vi "HandleObservationSync.vi"(8 "error in (no error)":errorcluster, 11 "S4GUI in":refnum<class "S4GUI.lvclass">) -> (0 "error out":errorcluster, 3 "S4GUI out":refnum<class "S4GUI.lvclass">)   [LabVIEW 2018, in "S4GUI.lvclass"] (continued)
          # "Espera terminar o envio de WAIT EXPOSE COMMAND para todos os ACS."
          n1279 = call-dynamic "VerifyAcqIdle.vi"("error in (no error)"=w3504, "S4GUI in"=w3503) -> ("error out"=w3509:errorcluster, "idle"=w3508:bool, "S4GUI out"=w3510:refnum<class "S4GUI.lvclass">)  [unwired: 6 in, 1 out]
          n1280 = disable-structure shown="Enabled" {
            disable-tunnel: w3506 -> [w3513 _]
            disable-tunnel: [w3512 u32 325] -> w3505
            frame Disabled {
              n1281 = Increment(x=w3513) -> (x+1=w3512:u32)
            }
            frame Enabled {
            }
          }
          n1282 = Select(t=w3505, s=w3508, f=w3506) -> (s? t:f=w3507:u32)
          n1283 = Bundle By Name(cluster=w3510, "Obs_state"=w3507) -> (w3511:refnum<class "S4GUI.lvclass">)
        }
        frame 323 {
          n1284 = call-dynamic "Read AcquisitionA.vi"("error in (no error)"=w3577, "S4ACS_GUI in"=w3578) -> ("error out"=w3532:errorcluster, "Acquisition.lvclass"=w3533:refnum<class "Acquisition.lvclass">, "S4ACS_GUI out"=w3580:refnum<class "S4GUI.lvclass">)  [unwired: 7 in]
          n1285 = call-dynamic "Read enabled.vi"("error in (no error)"=w3532, "Server in"=w3533) -> ("error out"=w3531:errorcluster, "enabled"=w3518:bool, "Server out"=w3534:refnum<class "Acquisition.lvclass">)  [unwired: 7 in]
          n1286 = call "Read connection.vi"("error in (no error)"=w3531, "Server in"=w3534) -> ("error out"=w3557:errorcluster, "connection"=w3541:bool, "Server out"=w3558:refnum<class "Acquisition.lvclass">)  [unwired: 7 in]
          n1287 = And(x=w3541, y=w3518) -> (x .and. y?=w3542:bool)
          n1288 = case shown="True" w3542 {
            tunnel: w3558 -> [w3687 w3703]
            tunnel: w3557 -> [w3686 w3702]
            tunnel: [w3687 w3700] -> w3581
            tunnel: [w3686 w3699] -> w3579
            tunnel: [w3683 u32 0 ("New_State")] -> w3547
            tunnel: w3518 -> [w3682 _]
            frame False {
              n1289 = Select(t=u32 1, s=w3682, f=u32 0) -> (s? t:f=w3683:u32)
            }
            frame True {
              n1290 = call-dynamic "Read Channel.vi"("error in (no error)"=w3702, "Acquisition in"=w3703) -> ("error out"=w3695:errorcluster, "Channel.lvclass"=w3694:refnum<class "Channel.lvclass">, "Acquisition out"=w3701:refnum<class "Acquisition.lvclass">)  [unwired: 7 in]
              n1291 = call-dynamic "Read State Machine.vi"("error in (no error)"=w3695, "Device in"=w3694) -> ("error out"=w3696:errorcluster, "State Machine.lvclass"=w3698:refnum<class "State Machine.lvclass">, "Device out"=w3692:refnum<class "Channel.lvclass">)  [unwired: 7 in]
              n1292 = call "Next State.vi"("error in (no error)"=w3696, "New_State"=50, "State Machine in"=w3698) -> ("error out"=w3689:errorcluster, "State Machine out"=w3690:refnum<class "State Machine.lvclass">)  [unwired: 7 in]
              n1293 = call-dynamic "Write State Machine.vi"("error in (no error)"=w3689, "State Machine.lvclass"=w3690, "Device in"=w3692) -> ("error out"=w3691:errorcluster, "Device out"=w3693:refnum<class "Channel.lvclass">)  [unwired: 7 in]
              n1294 = call-dynamic "Write Channel.vi"("error in (no error)"=w3691, "Channel.lvclass"=w3693, "Acquisition in"=w3701) -> ("error out"=w3699:errorcluster, "Acquisition out"=w3700:refnum<class "Acquisition.lvclass">)  [unwired: 7 in]
            }
          }
          n1295 = call-dynamic "Write AcquisitionA.vi"("error in (no error)"=w3579, "Acquisition.lvclass"=w3581, "S4ACS_GUI in"=w3580) -> ("error out"=w3574:errorcluster, "S4ACS_GUI out"=w3575:refnum<class "S4GUI.lvclass">)  [unwired: 7 in]
          n1296 = call "Read AcquisitionB.vi"("error in (no error)"=w3574, "S4ACS_GUI in"=w3575) -> ("error out"=w3528:errorcluster, "Acquisition.lvclass"=w3530:refnum<class "Acquisition.lvclass">, "S4ACS_GUI out"=w3572:refnum<class "S4GUI.lvclass">)  [unwired: 7 in]
          n1297 = call-dynamic "Read enabled.vi"("error in (no error)"=w3528, "Server in"=w3530) -> ("error out"=w3527:errorcluster, "enabled"=w3517:bool, "Server out"=w3529:refnum<class "Acquisition.lvclass">)  [unwired: 7 in]
          n1298 = call "Read connection.vi"("error in (no error)"=w3527, "Server in"=w3529) -> ("error out"=w3555:errorcluster, "connection"=w3539:bool, "Server out"=w3556:refnum<class "Acquisition.lvclass">)  [unwired: 7 in]
          n1299 = And(x=w3539, y=w3517) -> (x .and. y?=w3540:bool)
          n1300 = case shown="True" w3540 {
            tunnel: w3556 -> [w3665 w3681]
            tunnel: w3555 -> [w3664 w3680]
            tunnel: [w3665 w3678] -> w3573
            tunnel: [w3664 w3677] -> w3571
            tunnel: [w3661 u32 0 ("New_State")] -> w3546
            tunnel: w3517 -> [w3660 _]
            frame False {
              n1301 = Select(t=u32 2, s=w3660, f=u32 0) -> (s? t:f=w3661:u32)
            }
            frame True {
              n1302 = call-dynamic "Read Channel.vi"("error in (no error)"=w3680, "Acquisition in"=w3681) -> ("error out"=w3673:errorcluster, "Channel.lvclass"=w3672:refnum<class "Channel.lvclass">, "Acquisition out"=w3679:refnum<class "Acquisition.lvclass">)  [unwired: 7 in]
              n1303 = call-dynamic "Read State Machine.vi"("error in (no error)"=w3673, "Device in"=w3672) -> ("error out"=w3674:errorcluster, "State Machine.lvclass"=w3676:refnum<class "State Machine.lvclass">, "Device out"=w3670:refnum<class "Channel.lvclass">)  [unwired: 7 in]
              n1304 = call "Next State.vi"("error in (no error)"=w3674, "New_State"=50, "State Machine in"=w3676) -> ("error out"=w3667:errorcluster, "State Machine out"=w3668:refnum<class "State Machine.lvclass">)  [unwired: 7 in]
              n1305 = call-dynamic "Write State Machine.vi"("error in (no error)"=w3667, "State Machine.lvclass"=w3668, "Device in"=w3670) -> ("error out"=w3669:errorcluster, "Device out"=w3671:refnum<class "Channel.lvclass">)  [unwired: 7 in]
              n1306 = call-dynamic "Write Channel.vi"("error in (no error)"=w3669, "Channel.lvclass"=w3671, "Acquisition in"=w3679) -> ("error out"=w3677:errorcluster, "Acquisition out"=w3678:refnum<class "Acquisition.lvclass">)  [unwired: 7 in]
            }
          }
          n1307 = call "Write AcquisitionB.vi"("error in (no error)"=w3571, "Acquisition.lvclass"=w3573, "S4ACS_GUI in"=w3572) -> ("error out"=w3567:errorcluster, "S4ACS_GUI out"=w3566:refnum<class "S4GUI.lvclass">)  [unwired: 7 in]
          n1308 = call-dynamic "Read AcquisitionC.vi"("error in (no error)"=w3567, "S4ACS_GUI in"=w3566) -> ("error out"=w3524:errorcluster, "Acquisition.lvclass"=w3526:refnum<class "Acquisition.lvclass">, "S4ACS_GUI out"=w3569:refnum<class "S4GUI.lvclass">)  [unwired: 7 in]
          n1309 = call-dynamic "Read enabled.vi"("error in (no error)"=w3524, "Server in"=w3526) -> ("error out"=w3523:errorcluster, "enabled"=w3516:bool, "Server out"=w3525:refnum<class "Acquisition.lvclass">)  [unwired: 7 in]
          n1310 = call "Read connection.vi"("error in (no error)"=w3523, "Server in"=w3525) -> ("error out"=w3553:errorcluster, "connection"=w3536:bool, "Server out"=w3554:refnum<class "Acquisition.lvclass">)  [unwired: 7 in]
          n1311 = And(x=w3536, y=w3516) -> (x .and. y?=w3538:bool)
          n1312 = case shown="True" w3538 {
            tunnel: [w3642 w3651] -> w3570
            tunnel: [w3643 w3650] -> w3568
            tunnel: w3554 -> [w3643 w3648]
            tunnel: w3553 -> [w3642 w3647]
            tunnel: [w3639 u32 0 ("New_State")] -> w3545
            tunnel: w3516 -> [w3638 _]
            frame False {
              n1313 = Select(t=u32 4, s=w3638, f=u32 0) -> (s? t:f=w3639:u32)
            }
            frame True {
              n1314 = call-dynamic "Read Channel.vi"("error in (no error)"=w3647, "Acquisition in"=w3648) -> ("error out"=w3655:errorcluster, "Channel.lvclass"=w3656:refnum<class "Channel.lvclass">, "Acquisition out"=w3649:refnum<class "Acquisition.lvclass">)  [unwired: 7 in]
              n1315 = call-dynamic "Read State Machine.vi"("error in (no error)"=w3655, "Device in"=w3656) -> ("error out"=w3654:errorcluster, "State Machine.lvclass"=w3652:refnum<class "State Machine.lvclass">, "Device out"=w3658:refnum<class "Channel.lvclass">)  [unwired: 7 in]
              n1316 = call "Next State.vi"("error in (no error)"=w3654, "New_State"=50, "State Machine in"=w3652) -> ("error out"=w3646:errorcluster, "State Machine out"=w3645:refnum<class "State Machine.lvclass">)  [unwired: 7 in]
              n1317 = call-dynamic "Write State Machine.vi"("error in (no error)"=w3646, "State Machine.lvclass"=w3645, "Device in"=w3658) -> ("error out"=w3659:errorcluster, "Device out"=w3657:refnum<class "Channel.lvclass">)  [unwired: 7 in]
              n1318 = call-dynamic "Write Channel.vi"("error in (no error)"=w3659, "Channel.lvclass"=w3657, "Acquisition in"=w3649) -> ("error out"=w3651:errorcluster, "Acquisition out"=w3650:refnum<class "Acquisition.lvclass">)  [unwired: 7 in]
            }
          }
          n1319 = call-dynamic "Write AcquisitionC.vi"("error in (no error)"=w3570, "Acquisition.lvclass"=w3568, "S4ACS_GUI in"=w3569) -> ("error out"=w3564:errorcluster, "S4ACS_GUI out"=w3563:refnum<class "S4GUI.lvclass">)  [unwired: 7 in]
          n1320 = call-dynamic "Read AcquisitionD.vi"("error in (no error)"=w3564, "S4ACS_GUI in"=w3563) -> ("error out"=w3520:errorcluster, "Acquisition.lvclass"=w3522:refnum<class "Acquisition.lvclass">, "S4ACS_GUI out"=w3562:refnum<class "S4GUI.lvclass">)  [unwired: 7 in]
          n1321 = call-dynamic "Read enabled.vi"("error in (no error)"=w3520, "Server in"=w3522) -> ("error out"=w3519:errorcluster, "enabled"=w3515:bool, "Server out"=w3521:refnum<class "Acquisition.lvclass">)  [unwired: 7 in]
          n1322 = call "Read connection.vi"("error in (no error)"=w3519, "Server in"=w3521) -> ("error out"=w3551:errorcluster, "connection"=w3535:bool, "Server out"=w3552:refnum<class "Acquisition.lvclass">)  [unwired: 7 in]
          n1323 = And(x=w3535, y=w3515) -> (x .and. y?=w3537:bool)
          n1324 = case shown="True" w3537 {
            tunnel: w3551 -> [w3620 w3637]
            tunnel: [w3620 w3636] -> w3565
            tunnel: w3552 -> [w3621 w3627]
            tunnel: [w3621 w3625] -> w3561
            tunnel: [w3617 u32 0 ("New_State")] -> w3544
            tunnel: w3515 -> [w3616 _]
            frame False {
              n1325 = Select(t=u32 8, s=w3616, f=u32 0) -> (s? t:f=w3617:u32)
            }
            frame True {
              n1326 = call-dynamic "Read Channel.vi"("error in (no error)"=w3637, "Acquisition in"=w3627) -> ("error out"=w3632:errorcluster, "Channel.lvclass"=w3631:refnum<class "Channel.lvclass">, "Acquisition out"=w3626:refnum<class "Acquisition.lvclass">)  [unwired: 7 in]
              n1327 = call-dynamic "Read State Machine.vi"("error in (no error)"=w3632, "Device in"=w3631) -> ("error out"=w3633:errorcluster, "State Machine.lvclass"=w3635:refnum<class "State Machine.lvclass">, "Device out"=w3629:refnum<class "Channel.lvclass">)  [unwired: 7 in]
              n1328 = call "Next State.vi"("error in (no error)"=w3633, "New_State"=50, "State Machine in"=w3635) -> ("error out"=w3623:errorcluster, "State Machine out"=w3624:refnum<class "State Machine.lvclass">)  [unwired: 7 in]
              n1329 = call-dynamic "Write State Machine.vi"("error in (no error)"=w3623, "State Machine.lvclass"=w3624, "Device in"=w3629) -> ("error out"=w3628:errorcluster, "Device out"=w3630:refnum<class "Channel.lvclass">)  [unwired: 7 in]
              n1330 = call-dynamic "Write Channel.vi"("error in (no error)"=w3628, "Channel.lvclass"=w3630, "Acquisition in"=w3626) -> ("error out"=w3636:errorcluster, "Acquisition out"=w3625:refnum<class "Acquisition.lvclass">)  [unwired: 7 in]
            }
          }
          n1331 = call-dynamic "Write AcquisitionD.vi"("error in (no error)"=w3565, "Acquisition.lvclass"=w3561, "S4ACS_GUI in"=w3562) -> ("error out"=w3560:errorcluster, "S4ACS_GUI out"=w3559:refnum<class "S4GUI.lvclass">)  [unwired: 7 in]
          n1332 = Compound Arithmetic op=ADD(w3547, w3546, w3545, w3544) -> (w3548:u32)
          n1333 = case shown="0, Default" w3548 {
            tunnel: w3543 -> [w3585 _ _ _ _ _ _ _ _ _ _ _ _ _ _ _]
            tunnel: [w3584 u32 1 ("Obs_state") u32 1 ("Obs_state") u32 1 ("Obs_state") u32 1 ("Obs_state") u32 1 ("Obs_state") u32 1 ("Obs_state") u32 1 ("Obs_state") u32 1 ("Obs_state") u32 1 ("Obs_state") u32 1 ("Obs_state") u32 1 ("Obs_state") u32 1 ("Obs_state") u32 1 ("Obs_state") u32 1 ("Obs_state") u32 1 ("Obs_state")] -> w3549
            tunnel: ["" ("Error Msg") "ERROR: Lost channel 1 connection... - HandleObservationSync.vi state 323" ("Error Msg") "ERROR: Lost channel 2 connection...- HandleObservationSync.vi state 323" ("Error Msg") "ERROR: Lost channels 1 and 2 connection...- HandleObservationSync.vi state 323" ("Error Msg") "ERROR: Lost channel 3 connection...- HandleObservationSync.vi state 323" ("Error Msg") "ERROR: Lost channels 1 and  3 connection...- HandleObservationSync.vi state 323" ("Error Msg") "ERROR:  Lost channels 2 and  3 connection...- HandleObservationSync.vi state 323" ("Error Msg") "ERROR:  Lost channels 1, 2 and  3 connection...- HandleObservationSync.vi state 323" ("Error Msg") "ERROR: Lost channel 4 connection...- HandleObservationSync.vi state 323" ("Error Msg") "ERROR:  Lost channels 1 and 4 connection...- HandleObservationSync.vi state 323" ("Error Msg") "ERROR:  Lost channels 2 and 4 connection...- HandleObservationSync.vi state 323" ("Error Msg") "ERROR: Lost channels 1, 2 and 4 connection...- HandleObservationSync.vi state 323" ("Error Msg") "ERROR: Lost channels 3 and 4 connection...- HandleObservationSync.vi state 323" ("Error Msg") "ERROR: Lost channels 1, 3 and 4 connection...- HandleObservationSync.vi state 323" ("Error Msg") "ERROR: Lost channels 2, 3 and 4 connection...- HandleObservationSync.vi state 323" ("Error Msg") "ERROR: Lost channels 1, 2, 3 and 4 connection...- HandleObservationSync.vi state 323" ("Error Msg")] -> w3550
            frame 0, Default {
              n1334 = Increment(x=w3585) -> (x+1=w3584:u32)
              n1335 = Tick Count (ms)() -> (millisecond timer value=w3582:u32)
              n1336 = local write "time1"(w3582) -> ()
            }
            frame 1 {
            }
            frame 2 {
            }
            frame 3 {
            }
            frame 4 {
            }
            frame 5 {
            }
            frame 6 {
            }
            frame 7 {
            }
            frame 8 {
            }
            frame 9 {
            }
            frame 10 {
            }
            frame 11 {
            }
            frame 12 {
            }
            frame 13 {
            }
            frame 14 {
            }
            frame 15 {
            }
          }
          n1337 = Bundle By Name(cluster=w3559, "Obs_state"=w3549, "Error Msg"=w3550) -> (w3576:refnum<class "S4GUI.lvclass">)
        }
        frame 324 {
          # "Espera terminar a execução do comando atual \nantes de ir ao proximo passo da Observação."
          n1338 = call-dynamic "Read AcquisitionA.vi"("error in (no error)"=w3757, "S4ACS_GUI in"=w3758) -> ("error out"=w3739:errorcluster, "Acquisition.lvclass"=w3740:refnum<class "Acquisition.lvclass">, "S4ACS_GUI out"=w3760:refnum<class "S4GUI.lvclass">)  [unwired: 7 in]
          n1339 = call "Read connection.vi"("error in (no error)"=w3739, "Server in"=w3740) -> ("error out"=w3738:errorcluster, "connection"=w3737:bool, "Server out"=w3736:refnum<class "Acquisition.lvclass">)  [unwired: 7 in]
          n1340 = case shown="True" w3737 {
            tunnel: w3738 -> [w3869 w3890]
            tunnel: [w3870 w3888] -> w3761
            tunnel: [w3869 w3887] -> w3759
            tunnel: [TRUE w3876] -> w3718
            tunnel: w3736 -> [w3870 w3879]
            tunnel: [FALSE w3871] -> w3716
            frame False {
            }
            frame True {
              n1341 = call-dynamic "Read Channel.vi"("error in (no error)"=w3890, "Acquisition in"=w3879) -> ("error out"=w3873:errorcluster, "Channel.lvclass"=w3875:refnum<class "Channel.lvclass">, "Acquisition out"=w3889:refnum<class "Acquisition.lvclass">)  [unwired: 7 in]
              n1342 = call-dynamic "Read wait_expose.vi"("error in (no error)"=w3873, "Channel in"=w3875) -> ("error out"=w3872:errorcluster, "wait_expose"=w3871:bool, "Channel out"=w3874:refnum<class "Channel.lvclass">)  [unwired: 7 in]
              n1343 = call-dynamic "Read State Machine.vi"("error in (no error)"=w3872, "Device in"=w3874) -> ("error out"=w3881:errorcluster, "State Machine.lvclass"=w3883:refnum<class "State Machine.lvclass">, "Device out"=w3885:refnum<class "Channel.lvclass">)  [unwired: 7 in]
              n1344 = call-dynamic "Read State.vi"("error in (no error)"=w3881, "State Machine in"=w3883) -> ("error out"=w3880:errorcluster, "State"=w3877:i32, "State Machine out"=w3882:refnum<class "State Machine.lvclass">)  [unwired: 7 in]
              n1345 = Greater?(x=w3877, y=53 ("x")) -> (0:w3876:bool)
              n1346 = call-dynamic "Write State Machine.vi"("error in (no error)"=w3880, "State Machine.lvclass"=w3882, "Device in"=w3885) -> ("error out"=w3884:errorcluster, "Device out"=w3886:refnum<class "Channel.lvclass">)  [unwired: 7 in]
              n1347 = call-dynamic "Write Channel.vi"("error in (no error)"=w3884, "Channel.lvclass"=w3886, "Acquisition in"=w3889) -> ("error out"=w3887:errorcluster, "Acquisition out"=w3888:refnum<class "Acquisition.lvclass">)  [unwired: 7 in]
            }
          }
          n1348 = call-dynamic "Write AcquisitionA.vi"("error in (no error)"=w3759, "Acquisition.lvclass"=w3761, "S4ACS_GUI in"=w3760) -> ("error out"=w3754:errorcluster, "S4ACS_GUI out"=w3753:refnum<class "S4GUI.lvclass">)  [unwired: 7 in]
          n1349 = call "Read AcquisitionB.vi"("error in (no error)"=w3754, "S4ACS_GUI in"=w3753) -> ("error out"=w3731:errorcluster, "Acquisition.lvclass"=w3735:refnum<class "Acquisition.lvclass">, "S4ACS_GUI out"=w3755:refnum<class "S4GUI.lvclass">)  [unwired: 7 in]
          n1350 = call "Read connection.vi"("error in (no error)"=w3731, "Server in"=w3735) -> ("error out"=w3732:errorcluster, "connection"=w3733:bool, "Server out"=w3734:refnum<class "Acquisition.lvclass">)  [unwired: 7 in]
          n1351 = case shown="True" w3733 {
            tunnel: w3732 -> [w3845 w3858]
            tunnel: w3734 -> [w3846 w3857]
            tunnel: [TRUE w3852] -> w3720
            tunnel: [w3845 w3856] -> w3752
            tunnel: [w3846 w3855] -> w3751
            tunnel: [FALSE w3847] -> w3715
            frame False {
            }
            frame True {
              n1352 = call-dynamic "Read Channel.vi"("error in (no error)"=w3858, "Acquisition in"=w3857) -> ("error out"=w3849:errorcluster, "Channel.lvclass"=w3851:refnum<class "Channel.lvclass">, "Acquisition out"=w3859:refnum<class "Acquisition.lvclass">)  [unwired: 7 in]
              n1353 = call-dynamic "Read wait_expose.vi"("error in (no error)"=w3849, "Channel in"=w3851) -> ("error out"=w3848:errorcluster, "wait_expose"=w3847:bool, "Channel out"=w3850:refnum<class "Channel.lvclass">)  [unwired: 7 in]
              n1354 = call-dynamic "Read State Machine.vi"("error in (no error)"=w3848, "Device in"=w3850) -> ("error out"=w3865:errorcluster, "State Machine.lvclass"=w3863:refnum<class "State Machine.lvclass">, "Device out"=w3861:refnum<class "Channel.lvclass">)  [unwired: 7 in]
              n1355 = call-dynamic "Read State.vi"("error in (no error)"=w3865, "State Machine in"=w3863) -> ("error out"=w3866:errorcluster, "State"=w3854:i32, "State Machine out"=w3864:refnum<class "State Machine.lvclass">)  [unwired: 7 in]
              n1356 = Greater?(x=w3854, y=53 ("x")) -> (0:w3852:bool)
              n1357 = call-dynamic "Write State Machine.vi"("error in (no error)"=w3866, "State Machine.lvclass"=w3864, "Device in"=w3861) -> ("error out"=w3862:errorcluster, "Device out"=w3860:refnum<class "Channel.lvclass">)  [unwired: 7 in]
              n1358 = call-dynamic "Write Channel.vi"("error in (no error)"=w3862, "Channel.lvclass"=w3860, "Acquisition in"=w3859) -> ("error out"=w3856:errorcluster, "Acquisition out"=w3855:refnum<class "Acquisition.lvclass">)  [unwired: 7 in]
            }
          }
          n1359 = call "Write AcquisitionB.vi"("error in (no error)"=w3752, "Acquisition.lvclass"=w3751, "S4ACS_GUI in"=w3755) -> ("error out"=w3744:errorcluster, "S4ACS_GUI out"=w3743:refnum<class "S4GUI.lvclass">)  [unwired: 7 in]
          n1360 = call-dynamic "Read AcquisitionC.vi"("error in (no error)"=w3744, "S4ACS_GUI in"=w3743) -> ("error out"=w3727:errorcluster, "Acquisition.lvclass"=w3730:refnum<class "Acquisition.lvclass">, "S4ACS_GUI out"=w3746:refnum<class "S4GUI.lvclass">)  [unwired: 7 in]
          n1361 = call "Read connection.vi"("error in (no error)"=w3727, "Server in"=w3730) -> ("error out"=w3726:errorcluster, "connection"=w3728:bool, "Server out"=w3729:refnum<class "Acquisition.lvclass">)  [unwired: 7 in]
          n1362 = case shown="True" w3728 {
            tunnel: [w3821 w3835] -> w3747
            tunnel: [w3822 w3834] -> w3745
            tunnel: w3726 -> [w3821 w3831]
            tunnel: w3729 -> [w3822 w3832]
            tunnel: [TRUE w3828] -> w3719
            tunnel: [FALSE w3823] -> w3714
            frame False {
            }
            frame True {
              n1363 = call-dynamic "Read Channel.vi"("error in (no error)"=w3831, "Acquisition in"=w3832) -> ("error out"=w3825:errorcluster, "Channel.lvclass"=w3827:refnum<class "Channel.lvclass">, "Acquisition out"=w3833:refnum<class "Acquisition.lvclass">)  [unwired: 7 in]
              n1364 = call-dynamic "Read wait_expose.vi"("error in (no error)"=w3825, "Channel in"=w3827) -> ("error out"=w3824:errorcluster, "wait_expose"=w3823:bool, "Channel out"=w3826:refnum<class "Channel.lvclass">)  [unwired: 7 in]
              n1365 = call-dynamic "Read State Machine.vi"("error in (no error)"=w3824, "Device in"=w3826) -> ("error out"=w3841:errorcluster, "State Machine.lvclass"=w3839:refnum<class "State Machine.lvclass">, "Device out"=w3837:refnum<class "Channel.lvclass">)  [unwired: 7 in]
              n1366 = call-dynamic "Read State.vi"("error in (no error)"=w3841, "State Machine in"=w3839) -> ("error out"=w3842:errorcluster, "State"=w3829:i32, "State Machine out"=w3840:refnum<class "State Machine.lvclass">)  [unwired: 7 in]
              n1367 = Greater?(x=w3829, y=53 ("x")) -> (0:w3828:bool)
              n1368 = call-dynamic "Write State Machine.vi"("error in (no error)"=w3842, "State Machine.lvclass"=w3840, "Device in"=w3837) -> ("error out"=w3838:errorcluster, "Device out"=w3836:refnum<class "Channel.lvclass">)  [unwired: 7 in]
              n1369 = call-dynamic "Write Channel.vi"("error in (no error)"=w3838, "Channel.lvclass"=w3836, "Acquisition in"=w3833) -> ("error out"=w3835:errorcluster, "Acquisition out"=w3834:refnum<class "Acquisition.lvclass">)  [unwired: 7 in]
            }
          }
          n1370 = call-dynamic "Write AcquisitionC.vi"("error in (no error)"=w3747, "Acquisition.lvclass"=w3745, "S4ACS_GUI in"=w3746) -> ("error out"=w3741:errorcluster, "S4ACS_GUI out"=w3742:refnum<class "S4GUI.lvclass">)  [unwired: 7 in]
          n1371 = call-dynamic "Read AcquisitionD.vi"("error in (no error)"=w3741, "S4ACS_GUI in"=w3742) -> ("error out"=w3722:errorcluster, "Acquisition.lvclass"=w3725:refnum<class "Acquisition.lvclass">, "S4ACS_GUI out"=w3748:refnum<class "S4GUI.lvclass">)  [unwired: 7 in]
          n1372 = call "Read connection.vi"("error in (no error)"=w3722, "Server in"=w3725) -> ("error out"=w3721:errorcluster, "connection"=w3723:bool, "Server out"=w3724:refnum<class "Acquisition.lvclass">)  [unwired: 7 in]
          n1373 = case shown="True" w3723 {
            tunnel: [w3798 w3818] -> w3750
            tunnel: [w3797 w3817] -> w3749
            tunnel: w3724 -> [w3798 w3816]
            tunnel: w3721 -> [w3797 w3815]
            tunnel: [TRUE w3804] -> w3717
            tunnel: [FALSE w3799] -> w3713
            frame False {
            }
            frame True {
              n1374 = call-dynamic "Read Channel.vi"("error in (no error)"=w3815, "Acquisition in"=w3816) -> ("error out"=w3801:errorcluster, "Channel.lvclass"=w3803:refnum<class "Channel.lvclass">, "Acquisition out"=w3814:refnum<class "Acquisition.lvclass">)  [unwired: 7 in]
              n1375 = call-dynamic "Read wait_expose.vi"("error in (no error)"=w3801, "Channel in"=w3803) -> ("error out"=w3800:errorcluster, "wait_expose"=w3799:bool, "Channel out"=w3802:refnum<class "Channel.lvclass">)  [unwired: 7 in]
              n1376 = call-dynamic "Read State Machine.vi"("error in (no error)"=w3800, "Device in"=w3802) -> ("error out"=w3808:errorcluster, "State Machine.lvclass"=w3810:refnum<class "State Machine.lvclass">, "Device out"=w3812:refnum<class "Channel.lvclass">)  [unwired: 7 in]
              n1377 = call-dynamic "Read State.vi"("error in (no error)"=w3808, "State Machine in"=w3810) -> ("error out"=w3807:errorcluster, "State"=w3805:i32, "State Machine out"=w3809:refnum<class "State Machine.lvclass">)  [unwired: 7 in]
              n1378 = Greater?(x=w3805, y=53 ("x")) -> (0:w3804:bool)
              n1379 = call-dynamic "Write State Machine.vi"("error in (no error)"=w3807, "State Machine.lvclass"=w3809, "Device in"=w3812) -> ("error out"=w3811:errorcluster, "Device out"=w3813:refnum<class "Channel.lvclass">)  [unwired: 7 in]
              n1380 = call-dynamic "Write Channel.vi"("error in (no error)"=w3811, "Channel.lvclass"=w3813, "Acquisition in"=w3814) -> ("error out"=w3817:errorcluster, "Acquisition out"=w3818:refnum<class "Acquisition.lvclass">)  [unwired: 7 in]
            }
          }
          n1381 = call-dynamic "Write AcquisitionD.vi"("error in (no error)"=w3749, "Acquisition.lvclass"=w3750, "S4ACS_GUI in"=w3748) -> ("error out"=w3705:errorcluster, "S4ACS_GUI out"=w3708:refnum<class "S4GUI.lvclass">)  [unwired: 7 in]
          n1382 = Compound Arithmetic op=AND(w3718, w3720, w3719, w3717) -> (w3712:bool)
          n1383 = Compound Arithmetic op=OR(w3716, w3715, w3714, w3713) -> (w3710:bool)
          n1384 = call-dynamic "VerifErrors.vi"("error in (no error)"=w3705, "S4GUI in"=w3708) -> ("error out"=w3704:errorcluster, "Error value"=w3707:u32, "S4GUI out"=w3706:refnum<class "S4GUI.lvclass">)  [unwired: 7 in]
          n1385 = case shown="False" w3712 {
            tunnel: w3706 -> [w3764 w3794]
            tunnel: [w3770 w3793] -> w3709
            tunnel: w3711 -> [_ w3792]
            tunnel: w3710 -> [_ w3788]
            tunnel: w3707 -> [w3762 _]
            frame False {
              # "Aguardando iniciar exposição por 5s"
              n1386 = Tick Count (ms)() -> (millisecond timer value=w3769:u32)
              n1387 = local read "time1"() -> (w3763:u32)
              n1388 = Subtract(x=w3769, y=w3763) -> (x-y=w3766:u32)
              n1389 = To Double Precision Float(number=w3766) -> (double precision float=w3768:dbl)
              n1390 = Less?(x=5000.0 ("y"), y=w3768) -> (x < y?=w3767:bool)
              n1391 = case shown="False" w3767 {
                tunnel: w3764 -> [w3773 w3786]
                tunnel: [w3771 w3785] -> w3770
                tunnel: w3762 -> [w3772 _]
                frame False {
                  n1392 = case shown="1..15" w3772 {
                    selector: w3772 -> [_ w3781]
                    tunnel: [w3774 w3776] -> w3771
                    tunnel: w3773 -> [w3774 w3782]
                    frame 0, Default {
                    }
                    frame 1..15 {
                      n1393 = Number To Decimal String(number=w3781) -> (decimal integer string=w3778:string)  [unwired: 1 in]
                      n1394 = Concatenate Strings("CHANNEL ERROR <", w3778, ">: Error flag TRUE - see ACS panel.  HandleObservationSync.vi - state 324.") -> (w3780:string)
                      n1395 = Bundle By Name(cluster=w3782, "Obs_state"=u32 1, "Error Msg"=w3780) -> (w3776:refnum<class "S4GUI.lvclass">)
                    }
                  }
                }
                frame True {
                  n1396 = Bundle By Name(cluster=w3786, "Obs_state"=u32 1, "Error Msg"="ERROR: Acquisition Timeout. HandleObservationSync.vi - state 324.") -> (w3785:refnum<class "S4GUI.lvclass">)
                }
              }
            }
            frame True {
              # "327: Verifica incremento de ciclo."
              # "Iniciou aquisição..."
              n1397 = Increment(x=w3792) -> (x+1=w3789:u32)
              n1398 = Select(t=u32 327, s=w3788, f=w3789) -> (s? t:f=w3787:u32)
              n1399 = Tick Count (ms)() -> (millisecond timer value=w3791:u32)
              n1400 = Bundle By Name(cluster=w3794, "Obs_state"=w3787) -> (w3793:refnum<class "S4GUI.lvclass">)
              n1401 = local write "time307"(w3791) -> ()
            }
          }
          n1402 = Bundle By Name(cluster=w3709, "mode EXPOSE"=w3710) -> (w3756:refnum<class "S4GUI.lvclass">)
        }
        frame 325 {
          n1403 = Unbundle By Name(w3900) -> ("mode EXPOSE"=w3899:bool)
          n1404 = case shown="True" w3899 {
            tunnel: w3900 -> [w3953 w4020]
            tunnel: w3905 -> [w3952 w4019]
            tunnel: [w3951 w4017] -> w3904
            tunnel: [w3950 w4018] -> w3903
            tunnel: [w3949 w4016] -> w3893
            tunnel: w3901 -> [w3941 w4016]
            tunnel: [w3940 w3981] -> w3898
            tunnel: [w3940 w3980] -> w3897
            tunnel: [w3940 w3979] -> w3896
            tunnel: [w3940 w3978] -> w3895
            frame False {
              w3940 = 0
              n1405 = call-dynamic "Read Sync Box.lvclass.vi"("error in (no error)"=w3952, "SPARC4_AC in"=w3953) -> ("error out"=w3946:errorcluster, "Sync Box.lvclass"=w3948:refnum<class "Sync Box.lvclass">, "SPARC4_AC out"=w3943:refnum<class "S4GUI.lvclass">)  [unwired: 7 in]
              n1406 = call "Read connection.vi"("error in (no error)"=w3946, "Server in"=w3948) -> ("error out"=w3945:errorcluster, "connection"=w3944:bool, "Server out"=w3947:refnum<class "Sync Box.lvclass">)  [unwired: 7 in]
              n1407 = case shown="True" w3944 {
                tunnel: w3945 -> [w3959 w3977]
                tunnel: [w3960 w3975] -> w3955
                tunnel: [w3959 w3962] -> w3954
                tunnel: w3941 -> [w3956 w3961]
                tunnel: [w3958 w3961] -> w3949
                tunnel: w3947 -> [w3960 w3966]
                tunnel: w3943 -> [w3957 w3963]
                tunnel: [w3957 w3963] -> w3942
                frame False {
                  n1408 = Increment(x=w3956) -> (x+1=w3958:u32)
                }
                frame True {
                  # "Envia comando FIRE para o SyncBox"
                  n1409 = call-dynamic "Read Trigger.lvclass.vi"("error in (no error)"=w3977, "Sync Box in"=w3966) -> ("error out"=w3971:errorcluster, "Trigger.lvclass"=w3970:refnum<class "Trigger.lvclass">, "Sync Box out"=w3976:refnum<class "Sync Box.lvclass">)  [unwired: 7 in]
                  n1410 = call-dynamic "Read State Machine.vi"("error in (no error)"=w3971, "Device in"=w3970) -> ("error out"=w3972:errorcluster, "State Machine.lvclass"=w3974:refnum<class "State Machine.lvclass">, "Device out"=w3968:refnum<class "Trigger.lvclass">)  [unwired: 7 in]
                  n1411 = call "Next State.vi"("error in (no error)"=w3972, "New_State"=40, "State Machine in"=w3974) -> ("error out"=w3964:errorcluster, "State Machine out"=w3965:refnum<class "State Machine.lvclass">)  [unwired: 7 in]
                  n1412 = call-dynamic "Write State Machine.vi"("error in (no error)"=w3964, "State Machine.lvclass"=w3965, "Device in"=w3968) -> ("error out"=w3967:errorcluster, "Device out"=w3969:refnum<class "Trigger.lvclass">)  [unwired: 7 in]
                  n1413 = call-dynamic "Write Trigger.lvclass.vi"("error in (no error)"=w3967, "Trigger.lvclass"=w3969, "Sync Box in"=w3976) -> ("error out"=w3962:errorcluster, "Sync Box out"=w3975:refnum<class "Sync Box.lvclass">)  [unwired: 7 in]
                }
              }
              n1414 = call-dynamic "Write Sync Box.lvclass.vi"("error in (no error)"=w3954, "Sync Box.lvclass"=w3955, "SPARC4_AC in"=w3942) -> ("error out"=w3951:errorcluster, "SPARC4_AC out"=w3950:refnum<class "S4GUI.lvclass">)  [unwired: 7 in]
            }
            frame True {
              # "Envia comando EXPOSE para os canais ativos"
              n1415 = call-dynamic "Read AcquisitionA.vi"("error in (no error)"=w4019, "S4ACS_GUI in"=w4020) -> ("error out"=w4013:errorcluster, "Acquisition.lvclass"=w4015:refnum<class "Acquisition.lvclass">, "S4ACS_GUI out"=w4039:refnum<class "S4GUI.lvclass">)  [unwired: 7 in]
              n1416 = call-dynamic "Read enabled.vi"("error in (no error)"=w4013, "Server in"=w4015) -> ("error out"=w4012:errorcluster, "enabled"=w3985:bool, "Server out"=w4014:refnum<class "Acquisition.lvclass">)  [unwired: 7 in]
              n1417 = call "Read connection.vi"("error in (no error)"=w4012, "Server in"=w4014) -> ("error out"=w4021:errorcluster, "connection"=w4010:bool, "Server out"=w4022:refnum<class "Acquisition.lvclass">)  [unwired: 7 in]
              n1418 = And(x=w4010, y=w3985) -> (x .and. y?=w4011:bool)
              n1419 = case shown="False" w4011 {
                tunnel: w4022 -> [w4112 w4128]
                tunnel: w4021 -> [w4111 w4127]
                tunnel: [w4112 w4125] -> w4040
                tunnel: [w4111 w4124] -> w4038
                tunnel: [w4107 0] -> w3981
                tunnel: w3985 -> [w4108 _]
                frame False {
                  n1420 = Select(t=1, s=w4108, f=0) -> (s? t:f=w4107:i32)
                }
                frame True {
                  n1421 = call-dynamic "Read Channel.vi"("error in (no error)"=w4127, "Acquisition in"=w4128) -> ("error out"=w4120:errorcluster, "Channel.lvclass"=w4119:refnum<class "Channel.lvclass">, "Acquisition out"=w4126:refnum<class "Acquisition.lvclass">)  [unwired: 7 in]
                  n1422 = call-dynamic "Read State Machine.vi"("error in (no error)"=w4120, "Device in"=w4119) -> ("error out"=w4121:errorcluster, "State Machine.lvclass"=w4123:refnum<class "State Machine.lvclass">, "Device out"=w4117:refnum<class "Channel.lvclass">)  [unwired: 7 in]
                  n1423 = call "Next State.vi"("error in (no error)"=w4121, "New_State"=50, "State Machine in"=w4123) -> ("error out"=w4114:errorcluster, "State Machine out"=w4115:refnum<class "State Machine.lvclass">)  [unwired: 7 in]
                  n1424 = call-dynamic "Write State Machine.vi"("error in (no error)"=w4114, "State Machine.lvclass"=w4115, "Device in"=w4117) -> ("error out"=w4116:errorcluster, "Device out"=w4118:refnum<class "Channel.lvclass">)  [unwired: 7 in]
                  n1425 = call-dynamic "Write Channel.vi"("error in (no error)"=w4116, "Channel.lvclass"=w4118, "Acquisition in"=w4126) -> ("error out"=w4124:errorcluster, "Acquisition out"=w4125:refnum<class "Acquisition.lvclass">)  [unwired: 7 in]
                }
              }
              n1426 = call-dynamic "Write AcquisitionA.vi"("error in (no error)"=w4038, "Acquisition.lvclass"=w4040, "S4ACS_GUI in"=w4039) -> ("error out"=w4036:errorcluster, "S4ACS_GUI out"=w4037:refnum<class "S4GUI.lvclass">)  [unwired: 7 in]
              n1427 = call "Read AcquisitionB.vi"("error in (no error)"=w4036, "S4ACS_GUI in"=w4037) -> ("error out"=w4004:errorcluster, "Acquisition.lvclass"=w4006:refnum<class "Acquisition.lvclass">, "S4ACS_GUI out"=w4034:refnum<class "S4GUI.lvclass">)  [unwired: 7 in]
              n1428 = call-dynamic "Read enabled.vi"("error in (no error)"=w4004, "Server in"=w4006) -> ("error out"=w4008:errorcluster, "enabled"=w3984:bool, "Server out"=w4009:refnum<class "Acquisition.lvclass">)  [unwired: 7 in]
              n1429 = call "Read connection.vi"("error in (no error)"=w4008, "Server in"=w4009) -> ("error out"=w4003:errorcluster, "connection"=w4007:bool, "Server out"=w4005:refnum<class "Acquisition.lvclass">)  [unwired: 7 in]
              n1430 = And(x=w4007, y=w3984) -> (x .and. y?=w4002:bool)
              n1431 = case shown="True" w4002 {
                tunnel: w4005 -> [w4090 w4106]
                tunnel: w4003 -> [w4089 w4105]
                tunnel: [w4090 w4103] -> w4035
                tunnel: [w4089 w4102] -> w4033
                tunnel: [w4086 0] -> w3980
                tunnel: w3984 -> [w4085 _]
                frame False {
                  n1432 = Select(t=2, s=w4085, f=0) -> (s? t:f=w4086:i32)
                }
                frame True {
                  n1433 = call-dynamic "Read Channel.vi"("error in (no error)"=w4105, "Acquisition in"=w4106) -> ("error out"=w4098:errorcluster, "Channel.lvclass"=w4097:refnum<class "Channel.lvclass">, "Acquisition out"=w4104:refnum<class "Acquisition.lvclass">)  [unwired: 7 in]
                  n1434 = call-dynamic "Read State Machine.vi"("error in (no error)"=w4098, "Device in"=w4097) -> ("error out"=w4099:errorcluster, "State Machine.lvclass"=w4101:refnum<class "State Machine.lvclass">, "Device out"=w4095:refnum<class "Channel.lvclass">)  [unwired: 7 in]
                  n1435 = call "Next State.vi"("error in (no error)"=w4099, "New_State"=50, "State Machine in"=w4101) -> ("error out"=w4092:errorcluster, "State Machine out"=w4093:refnum<class "State Machine.lvclass">)  [unwired: 7 in]
                  n1436 = call-dynamic "Write State Machine.vi"("error in (no error)"=w4092, "State Machine.lvclass"=w4093, "Device in"=w4095) -> ("error out"=w4094:errorcluster, "Device out"=w4096:refnum<class "Channel.lvclass">)  [unwired: 7 in]
                  n1437 = call-dynamic "Write Channel.vi"("error in (no error)"=w4094, "Channel.lvclass"=w4096, "Acquisition in"=w4104) -> ("error out"=w4102:errorcluster, "Acquisition out"=w4103:refnum<class "Acquisition.lvclass">)  [unwired: 7 in]
                }
              }
              n1438 = call "Write AcquisitionB.vi"("error in (no error)"=w4033, "Acquisition.lvclass"=w4035, "S4ACS_GUI in"=w4034) -> ("error out"=w4029:errorcluster, "S4ACS_GUI out"=w4028:refnum<class "S4GUI.lvclass">)  [unwired: 7 in]
              n1439 = call-dynamic "Read AcquisitionC.vi"("error in (no error)"=w4029, "S4ACS_GUI in"=w4028) -> ("error out"=w3995:errorcluster, "Acquisition.lvclass"=w3996:refnum<class "Acquisition.lvclass">, "S4ACS_GUI out"=w4031:refnum<class "S4GUI.lvclass">)  [unwired: 7 in]
              n1440 = call-dynamic "Read enabled.vi"("error in (no error)"=w3995, "Server in"=w3996) -> ("error out"=w4000:errorcluster, "enabled"=w3983:bool, "Server out"=w4001:refnum<class "Acquisition.lvclass">)  [unwired: 7 in]
              n1441 = call "Read connection.vi"("error in (no error)"=w4000, "Server in"=w4001) -> ("error out"=w3997:errorcluster, "connection"=w3999:bool, "Server out"=w3998:refnum<class "Acquisition.lvclass">)  [unwired: 7 in]
              n1442 = And(x=w3999, y=w3983) -> (x .and. y?=w3994:bool)
              n1443 = case shown="False" w3994 {
                tunnel: [w4067 w4076] -> w4032
                tunnel: [w4068 w4075] -> w4030
                tunnel: w3998 -> [w4068 w4073]
                tunnel: w3997 -> [w4067 w4072]
                tunnel: [w4063 0] -> w3979
                tunnel: w3983 -> [w4064 _]
                frame False {
                  n1444 = Select(t=4, s=w4064, f=0) -> (s? t:f=w4063:i32)
                }
                frame True {
                  n1445 = call-dynamic "Read Channel.vi"("error in (no error)"=w4072, "Acquisition in"=w4073) -> ("error out"=w4080:errorcluster, "Channel.lvclass"=w4081:refnum<class "Channel.lvclass">, "Acquisition out"=w4074:refnum<class "Acquisition.lvclass">)  [unwired: 7 in]
                  n1446 = call-dynamic "Read State Machine.vi"("error in (no error)"=w4080, "Device in"=w4081) -> ("error out"=w4079:errorcluster, "State Machine.lvclass"=w4077:refnum<class "State Machine.lvclass">, "Device out"=w4083:refnum<class "Channel.lvclass">)  [unwired: 7 in]
                  n1447 = call "Next State.vi"("error in (no error)"=w4079, "New_State"=50, "State Machine in"=w4077) -> ("error out"=w4071:errorcluster, "State Machine out"=w4070:refnum<class "State Machine.lvclass">)  [unwired: 7 in]
                  n1448 = call-dynamic "Write State Machine.vi"("error in (no error)"=w4071, "State Machine.lvclass"=w4070, "Device in"=w4083) -> ("error out"=w4084:errorcluster, "Device out"=w4082:refnum<class "Channel.lvclass">)  [unwired: 7 in]
                  n1449 = call-dynamic "Write Channel.vi"("error in (no error)"=w4084, "Channel.lvclass"=w4082, "Acquisition in"=w4074) -> ("error out"=w4076:errorcluster, "Acquisition out"=w4075:refnum<class "Acquisition.lvclass">)  [unwired: 7 in]
                }
              }
              n1450 = call-dynamic "Write AcquisitionC.vi"("error in (no error)"=w4032, "Acquisition.lvclass"=w4030, "S4ACS_GUI in"=w4031) -> ("error out"=w4026:errorcluster, "S4ACS_GUI out"=w4025:refnum<class "S4GUI.lvclass">)  [unwired: 7 in]
              n1451 = call-dynamic "Read AcquisitionD.vi"("error in (no error)"=w4026, "S4ACS_GUI in"=w4025) -> ("error out"=w3987:errorcluster, "Acquisition.lvclass"=w3988:refnum<class "Acquisition.lvclass">, "S4ACS_GUI out"=w4024:refnum<class "S4GUI.lvclass">)  [unwired: 7 in]
              n1452 = call-dynamic "Read enabled.vi"("error in (no error)"=w3987, "Server in"=w3988) -> ("error out"=w3992:errorcluster, "enabled"=w3982:bool, "Server out"=w3993:refnum<class "Acquisition.lvclass">)  [unwired: 7 in]
              n1453 = call "Read connection.vi"("error in (no error)"=w3992, "Server in"=w3993) -> ("error out"=w3990:errorcluster, "connection"=w3991:bool, "Server out"=w3989:refnum<class "Acquisition.lvclass">)  [unwired: 7 in]
              n1454 = And(x=w3991, y=w3982) -> (x .and. y?=w3986:bool)
              n1455 = case shown="False" w3986 {
                tunnel: w3990 -> [w4045 w4062]
                tunnel: [w4045 w4061] -> w4027
                tunnel: w3989 -> [w4046 w4052]
                tunnel: [w4046 w4050] -> w4023
                tunnel: [w4041 0] -> w3978
                tunnel: w3982 -> [w4042 _]
                frame False {
                  n1456 = Select(t=8, s=w4042, f=0) -> (s? t:f=w4041:i32)
                }
                frame True {
                  n1457 = call-dynamic "Read Channel.vi"("error in (no error)"=w4062, "Acquisition in"=w4052) -> ("error out"=w4057:errorcluster, "Channel.lvclass"=w4056:refnum<class "Channel.lvclass">, "Acquisition out"=w4051:refnum<class "Acquisition.lvclass">)  [unwired: 7 in]
                  n1458 = call-dynamic "Read State Machine.vi"("error in (no error)"=w4057, "Device in"=w4056) -> ("error out"=w4058:errorcluster, "State Machine.lvclass"=w4060:refnum<class "State Machine.lvclass">, "Device out"=w4054:refnum<class "Channel.lvclass">)  [unwired: 7 in]
                  n1459 = call "Next State.vi"("error in (no error)"=w4058, "New_State"=50, "State Machine in"=w4060) -> ("error out"=w4048:errorcluster, "State Machine out"=w4049:refnum<class "State Machine.lvclass">)  [unwired: 7 in]
                  n1460 = call-dynamic "Write State Machine.vi"("error in (no error)"=w4048, "State Machine.lvclass"=w4049, "Device in"=w4054) -> ("error out"=w4053:errorcluster, "Device out"=w4055:refnum<class "Channel.lvclass">)  [unwired: 7 in]
                  n1461 = call-dynamic "Write Channel.vi"("error in (no error)"=w4053, "Channel.lvclass"=w4055, "Acquisition in"=w4051) -> ("error out"=w4061:errorcluster, "Acquisition out"=w4050:refnum<class "Acquisition.lvclass">)  [unwired: 7 in]
                }
              }
              n1462 = call-dynamic "Write AcquisitionD.vi"("error in (no error)"=w4027, "Acquisition.lvclass"=w4023, "S4ACS_GUI in"=w4024) -> ("error out"=w4017:errorcluster, "S4ACS_GUI out"=w4018:refnum<class "S4GUI.lvclass">)  [unwired: 7 in]
            }
          }
          n1463 = Compound Arithmetic op=ADD(w3898, w3897, w3896, w3895) -> (w3894:i32)
          n1464 = case shown="0, Default" w3894 {
            tunnel: w3893 -> [w3909 _ _ _ _ _ _ _ _ _ _ _ _ _ _ _]
            tunnel: [w3908 u32 1 ("Obs_state") u32 1 ("Obs_state") u32 1 ("Obs_state") u32 1 ("Obs_state") u32 1 ("Obs_state") u32 1 ("Obs_state") u32 1 ("Obs_state") u32 1 ("Obs_state") u32 1 ("Obs_state") u32 1 ("Obs_state") u32 1 ("Obs_state") u32 1 ("Obs_state") u32 1 ("Obs_state") u32 1 ("Obs_state") u32 1 ("Obs_state")] -> w3892
            tunnel: ["" ("Error Msg") "ERROR: Lost channel 1 connection... - HandleObservationSync.vi state 325" ("Error Msg") "ERROR: Lost channel 2 connection...- HandleObservationSync.vi state 325" ("Error Msg") "ERROR: Lost channels 1 and 2 connection...- HandleObservationSync.vi state 325" ("Error Msg") "ERROR: Lost channel 3 connection...- HandleObservationSync.vi state 325" ("Error Msg") "ERROR: Lost channels 1 and  3 connection...- HandleObservationSync.vi state 325" ("Error Msg") "ERROR:  Lost channels 2 and  3 connection...- HandleObservationSync.vi state 325" ("Error Msg") "ERROR:  Lost channels 1, 2 and  3 connection...- HandleObservationSync.vi state 325" ("Error Msg") "ERROR: Lost channel 4 connection...- HandleObservationSync.vi state 325" ("Error Msg") "ERROR:  Lost channels 1 and 4 connection...- HandleObservationSync.vi state 325" ("Error Msg") "ERROR:  Lost channels 2 and 4 connection...- HandleObservationSync.vi state 325" ("Error Msg") "ERROR: Lost channels 1, 2 and 4 connection...- HandleObservationSync.vi state 325" ("Error Msg") "ERROR: Lost channels 3 and 4 connection...- HandleObservationSync.vi state 325" ("Error Msg") "ERROR: Lost channels 1, 3 and 4 connection...- HandleObservationSync.vi state 325" ("Error Msg") "ERROR: Lost channels 2, 3 and 4 connection...- HandleObservationSync.vi state 325" ("Error Msg") "ERROR: Lost channels 1, 2, 3 and 4 connection...- HandleObservationSync.vi state 325" ("Error Msg")] -> w3891
            frame 0, Default {
              n1465 = Increment(x=w3909) -> (x+1=w3908:u32)
              n1466 = Tick Count (ms)() -> (millisecond timer value=w3906:u32)
              n1467 = local write "time1"(w3906) -> ()
            }
            frame 1 {
            }
            frame 2 {
            }
            frame 3 {
            }
            frame 4 {
            }
            frame 5 {
            }
            frame 6 {
            }
            frame 7 {
            }
            frame 8 {
            }
            frame 9 {
            }
            frame 10 {
            }
            frame 11 {
            }
            frame 12 {
            }
            frame 13 {
            }
            frame 14 {
            }
            frame 15 {
            }
          }
          n1468 = Bundle By Name(cluster=w3903, "Obs_state"=w3892, "Error Msg"=w3891) -> (w3902:refnum<class "S4GUI.lvclass">)
        }
        frame 326 {
          # "Espera terminar a execução do comando atual \nantes de ir ao proximo passo da Observação."
          n1469 = call-dynamic "Read AcquisitionA.vi"("error in (no error)"=w4182, "S4ACS_GUI in"=w4183) -> ("error out"=w4164:errorcluster, "Acquisition.lvclass"=w4165:refnum<class "Acquisition.lvclass">, "S4ACS_GUI out"=w4185:refnum<class "S4GUI.lvclass">)  [unwired: 7 in]
          n1470 = call "Read connection.vi"("error in (no error)"=w4164, "Server in"=w4165) -> ("error out"=w4163:errorcluster, "connection"=w4162:bool, "Server out"=w4161:refnum<class "Acquisition.lvclass">)  [unwired: 7 in]
          n1471 = case shown="False" w4162 {
            tunnel: w4163 -> [w4284 w4305]
            tunnel: [w4285 w4303] -> w4186
            tunnel: [w4284 w4302] -> w4184
            tunnel: [TRUE w4291] -> w4143
            tunnel: w4161 -> [w4285 w4294]
            tunnel: [FALSE w4286] -> w4141
            frame False {
            }
            frame True {
              n1472 = call-dynamic "Read Channel.vi"("error in (no error)"=w4305, "Acquisition in"=w4294) -> ("error out"=w4288:errorcluster, "Channel.lvclass"=w4290:refnum<class "Channel.lvclass">, "Acquisition out"=w4304:refnum<class "Acquisition.lvclass">)  [unwired: 7 in]
              n1473 = call-dynamic "Read wait_expose.vi"("error in (no error)"=w4288, "Channel in"=w4290) -> ("error out"=w4287:errorcluster, "wait_expose"=w4286:bool, "Channel out"=w4289:refnum<class "Channel.lvclass">)  [unwired: 7 in]
              n1474 = call-dynamic "Read State Machine.vi"("error in (no error)"=w4287, "Device in"=w4289) -> ("error out"=w4296:errorcluster, "State Machine.lvclass"=w4298:refnum<class "State Machine.lvclass">, "Device out"=w4300:refnum<class "Channel.lvclass">)  [unwired: 7 in]
              n1475 = call-dynamic "Read State.vi"("error in (no error)"=w4296, "State Machine in"=w4298) -> ("error out"=w4295:errorcluster, "State"=w4292:i32, "State Machine out"=w4297:refnum<class "State Machine.lvclass">)  [unwired: 7 in]
              n1476 = Greater?(x=w4292, y=53 ("x")) -> (0:w4291:bool)
              n1477 = call-dynamic "Write State Machine.vi"("error in (no error)"=w4295, "State Machine.lvclass"=w4297, "Device in"=w4300) -> ("error out"=w4299:errorcluster, "Device out"=w4301:refnum<class "Channel.lvclass">)  [unwired: 7 in]
              n1478 = call-dynamic "Write Channel.vi"("error in (no error)"=w4299, "Channel.lvclass"=w4301, "Acquisition in"=w4304) -> ("error out"=w4302:errorcluster, "Acquisition out"=w4303:refnum<class "Acquisition.lvclass">)  [unwired: 7 in]
            }
          }
          n1479 = call-dynamic "Write AcquisitionA.vi"("error in (no error)"=w4184, "Acquisition.lvclass"=w4186, "S4ACS_GUI in"=w4185) -> ("error out"=w4179:errorcluster, "S4ACS_GUI out"=w4178:refnum<class "S4GUI.lvclass">)  [unwired: 7 in]
          n1480 = call "Read AcquisitionB.vi"("error in (no error)"=w4179, "S4ACS_GUI in"=w4178) -> ("error out"=w4156:errorcluster, "Acquisition.lvclass"=w4160:refnum<class "Acquisition.lvclass">, "S4ACS_GUI out"=w4180:refnum<class "S4GUI.lvclass">)  [unwired: 7 in]
          n1481 = call "Read connection.vi"("error in (no error)"=w4156, "Server in"=w4160) -> ("error out"=w4157:errorcluster, "connection"=w4158:bool, "Server out"=w4159:refnum<class "Acquisition.lvclass">)  [unwired: 7 in]
          n1482 = case shown="True" w4158 {
            tunnel: w4157 -> [w4260 w4273]
            tunnel: w4159 -> [w4261 w4272]
            tunnel: [TRUE w4267] -> w4145
            tunnel: [w4260 w4271] -> w4177
            tunnel: [w4261 w4270] -> w4176
            tunnel: [FALSE w4262] -> w4140
            frame False {
            }
            frame True {
              n1483 = call-dynamic "Read Channel.vi"("error in (no error)"=w4273, "Acquisition in"=w4272) -> ("error out"=w4264:errorcluster, "Channel.lvclass"=w4266:refnum<class "Channel.lvclass">, "Acquisition out"=w4274:refnum<class "Acquisition.lvclass">)  [unwired: 7 in]
              n1484 = call-dynamic "Read wait_expose.vi"("error in (no error)"=w4264, "Channel in"=w4266) -> ("error out"=w4263:errorcluster, "wait_expose"=w4262:bool, "Channel out"=w4265:refnum<class "Channel.lvclass">)  [unwired: 7 in]
              n1485 = call-dynamic "Read State Machine.vi"("error in (no error)"=w4263, "Device in"=w4265) -> ("error out"=w4280:errorcluster, "State Machine.lvclass"=w4278:refnum<class "State Machine.lvclass">, "Device out"=w4276:refnum<class "Channel.lvclass">)  [unwired: 7 in]
              n1486 = call-dynamic "Read State.vi"("error in (no error)"=w4280, "State Machine in"=w4278) -> ("error out"=w4281:errorcluster, "State"=w4269:i32, "State Machine out"=w4279:refnum<class "State Machine.lvclass">)  [unwired: 7 in]
              n1487 = Greater?(x=w4269, y=53 ("x")) -> (0:w4267:bool)
              n1488 = call-dynamic "Write State Machine.vi"("error in (no error)"=w4281, "State Machine.lvclass"=w4279, "Device in"=w4276) -> ("error out"=w4277:errorcluster, "Device out"=w4275:refnum<class "Channel.lvclass">)  [unwired: 7 in]
              n1489 = call-dynamic "Write Channel.vi"("error in (no error)"=w4277, "Channel.lvclass"=w4275, "Acquisition in"=w4274) -> ("error out"=w4271:errorcluster, "Acquisition out"=w4270:refnum<class "Acquisition.lvclass">)  [unwired: 7 in]
            }
          }
          n1490 = call "Write AcquisitionB.vi"("error in (no error)"=w4177, "Acquisition.lvclass"=w4176, "S4ACS_GUI in"=w4180) -> ("error out"=w4169:errorcluster, "S4ACS_GUI out"=w4168:refnum<class "S4GUI.lvclass">)  [unwired: 7 in]
          n1491 = call-dynamic "Read AcquisitionC.vi"("error in (no error)"=w4169, "S4ACS_GUI in"=w4168) -> ("error out"=w4152:errorcluster, "Acquisition.lvclass"=w4155:refnum<class "Acquisition.lvclass">, "S4ACS_GUI out"=w4171:refnum<class "S4GUI.lvclass">)  [unwired: 7 in]
          n1492 = call "Read connection.vi"("error in (no error)"=w4152, "Server in"=w4155) -> ("error out"=w4151:errorcluster, "connection"=w4153:bool, "Server out"=w4154:refnum<class "Acquisition.lvclass">)  [unwired: 7 in]
          n1493 = case shown="True" w4153 {
            tunnel: [w4236 w4250] -> w4172
            tunnel: [w4237 w4249] -> w4170
            tunnel: w4151 -> [w4236 w4246]
            tunnel: w4154 -> [w4237 w4247]
            tunnel: [TRUE w4243] -> w4144
            tunnel: [FALSE w4238] -> w4139
            frame False {
            }
            frame True {
              n1494 = call-dynamic "Read Channel.vi"("error in (no error)"=w4246, "Acquisition in"=w4247) -> ("error out"=w4240:errorcluster, "Channel.lvclass"=w4242:refnum<class "Channel.lvclass">, "Acquisition out"=w4248:refnum<class "Acquisition.lvclass">)  [unwired: 7 in]
              n1495 = call-dynamic "Read wait_expose.vi"("error in (no error)"=w4240, "Channel in"=w4242) -> ("error out"=w4239:errorcluster, "wait_expose"=w4238:bool, "Channel out"=w4241:refnum<class "Channel.lvclass">)  [unwired: 7 in]
              n1496 = call-dynamic "Read State Machine.vi"("error in (no error)"=w4239, "Device in"=w4241) -> ("error out"=w4256:errorcluster, "State Machine.lvclass"=w4254:refnum<class "State Machine.lvclass">, "Device out"=w4252:refnum<class "Channel.lvclass">)  [unwired: 7 in]
              n1497 = call-dynamic "Read State.vi"("error in (no error)"=w4256, "State Machine in"=w4254) -> ("error out"=w4257:errorcluster, "State"=w4244:i32, "State Machine out"=w4255:refnum<class "State Machine.lvclass">)  [unwired: 7 in]
              n1498 = Greater?(x=w4244, y=53 ("x")) -> (0:w4243:bool)
              n1499 = call-dynamic "Write State Machine.vi"("error in (no error)"=w4257, "State Machine.lvclass"=w4255, "Device in"=w4252) -> ("error out"=w4253:errorcluster, "Device out"=w4251:refnum<class "Channel.lvclass">)  [unwired: 7 in]
              n1500 = call-dynamic "Write Channel.vi"("error in (no error)"=w4253, "Channel.lvclass"=w4251, "Acquisition in"=w4248) -> ("error out"=w4250:errorcluster, "Acquisition out"=w4249:refnum<class "Acquisition.lvclass">)  [unwired: 7 in]
            }
          }
          n1501 = call-dynamic "Write AcquisitionC.vi"("error in (no error)"=w4172, "Acquisition.lvclass"=w4170, "S4ACS_GUI in"=w4171) -> ("error out"=w4166:errorcluster, "S4ACS_GUI out"=w4167:refnum<class "S4GUI.lvclass">)  [unwired: 7 in]
          n1502 = call-dynamic "Read AcquisitionD.vi"("error in (no error)"=w4166, "S4ACS_GUI in"=w4167) -> ("error out"=w4147:errorcluster, "Acquisition.lvclass"=w4150:refnum<class "Acquisition.lvclass">, "S4ACS_GUI out"=w4173:refnum<class "S4GUI.lvclass">)  [unwired: 7 in]
          n1503 = call "Read connection.vi"("error in (no error)"=w4147, "Server in"=w4150) -> ("error out"=w4146:errorcluster, "connection"=w4148:bool, "Server out"=w4149:refnum<class "Acquisition.lvclass">)  [unwired: 7 in]
          n1504 = case shown="True" w4148 {
            tunnel: [w4213 w4233] -> w4175
            tunnel: [w4212 w4232] -> w4174
            tunnel: w4149 -> [w4213 w4231]
            tunnel: w4146 -> [w4212 w4230]
            tunnel: [TRUE w4219] -> w4142
            tunnel: [FALSE w4214] -> w4138
            frame False {
            }
            frame True {
              n1505 = call-dynamic "Read Channel.vi"("error in (no error)"=w4230, "Acquisition in"=w4231) -> ("error out"=w4216:errorcluster, "Channel.lvclass"=w4218:refnum<class "Channel.lvclass">, "Acquisition out"=w4229:refnum<class "Acquisition.lvclass">)  [unwired: 7 in]
              n1506 = call-dynamic "Read wait_expose.vi"("error in (no error)"=w4216, "Channel in"=w4218) -> ("error out"=w4215:errorcluster, "wait_expose"=w4214:bool, "Channel out"=w4217:refnum<class "Channel.lvclass">)  [unwired: 7 in]
              n1507 = call-dynamic "Read State Machine.vi"("error in (no error)"=w4215, "Device in"=w4217) -> ("error out"=w4223:errorcluster, "State Machine.lvclass"=w4225:refnum<class "State Machine.lvclass">, "Device out"=w4227:refnum<class "Channel.lvclass">)  [unwired: 7 in]
              n1508 = call-dynamic "Read State.vi"("error in (no error)"=w4223, "State Machine in"=w4225) -> ("error out"=w4222:errorcluster, "State"=w4220:i32, "State Machine out"=w4224:refnum<class "State Machine.lvclass">)  [unwired: 7 in]
              n1509 = Greater?(x=w4220, y=53 ("x")) -> (0:w4219:bool)
              n1510 = call-dynamic "Write State Machine.vi"("error in (no error)"=w4222, "State Machine.lvclass"=w4224, "Device in"=w4227) -> ("error out"=w4226:errorcluster, "Device out"=w4228:refnum<class "Channel.lvclass">)  [unwired: 7 in]
              n1511 = call-dynamic "Write Channel.vi"("error in (no error)"=w4226, "Channel.lvclass"=w4228, "Acquisition in"=w4229) -> ("error out"=w4232:errorcluster, "Acquisition out"=w4233:refnum<class "Acquisition.lvclass">)  [unwired: 7 in]
            }
          }
          n1512 = call-dynamic "Write AcquisitionD.vi"("error in (no error)"=w4174, "Acquisition.lvclass"=w4175, "S4ACS_GUI in"=w4173) -> ("error out"=w4131:errorcluster, "S4ACS_GUI out"=w4133:refnum<class "S4GUI.lvclass">)  [unwired: 7 in]
          n1513 = Compound Arithmetic op=AND(w4143, w4145, w4144, w4142) -> (w4136:bool)
          n1514 = Compound Arithmetic op=OR(w4141, w4140, w4139, w4138) -> (w4137:bool)
          n1515 = call-dynamic "VerifErrors.vi"("error in (no error)"=w4131, "S4GUI in"=w4133) -> ("error out"=w4130:errorcluster, "Error value"=w4129:u32, "S4GUI out"=w4132:refnum<class "S4GUI.lvclass">)  [unwired: 7 in]
          n1516 = case shown="False" w4136 {
